vi "ROI entry-Previous ROI compat-planes.vi"(8 "error in (no error)":errorcluster, 9 "Proceed":bool=TRUE, 11 "Old ROI file path":path) -> (0 "error out":errorcluster, 1 "Proceed":bool, 3 "Old ROI file path (dup)":path)   [LabVIEW 2013]
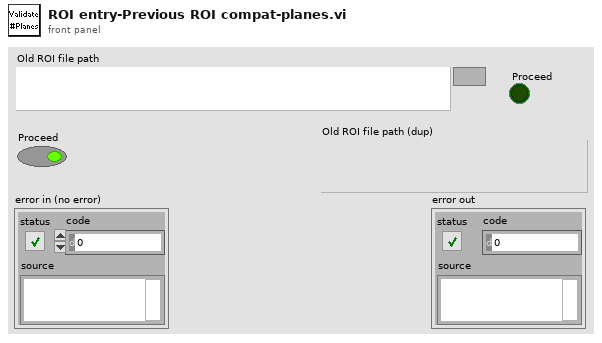
[diagram p1: front panel]
types:
  T1 = typedef "Fixed strings.ctl" = cluster{"ROI file name":string, "Normalised ROI file name":string, "Zplane Pockels values file name":string, "Functional data folder name":string, "Experiment Header file name":string, "Z-stack images folder name":string, "Groups setup rel. path":string, "Groups text file rel. path":string, "TDMS files folder name (F.img)":string, "TDMS files folder name (V.acq)":string, "TDMS files folder name (Pl.acq)":string, "Cycle rel times sequence file":string, "Dynamically called VIs folder name":string, "Time Series folder base name":string}
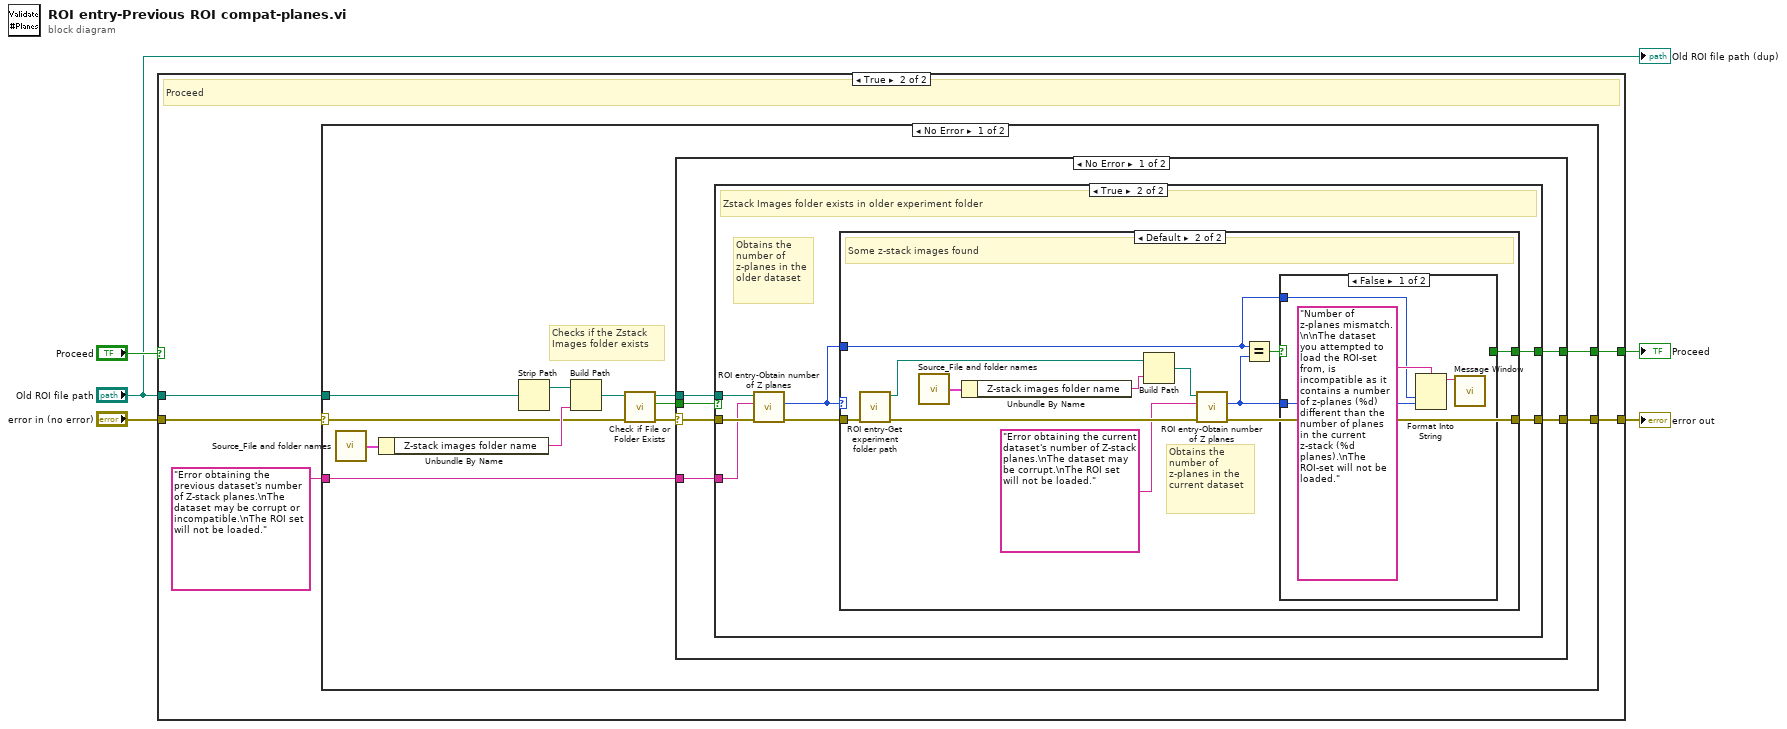
[diagram p0: block diagram]
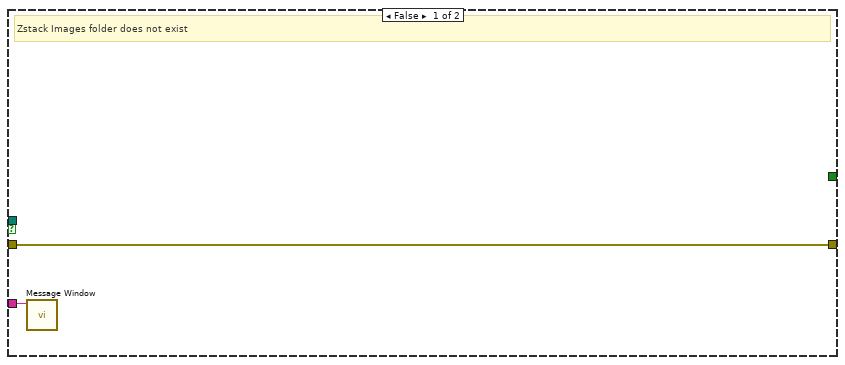
[diagram p3: hidden frame]
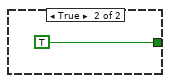
[diagram p5: hidden frame]
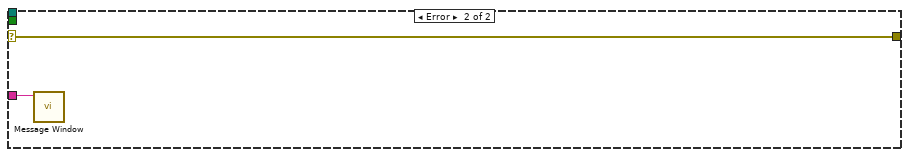
[diagram p6: hidden frame]
diagram:
  n1 = case shown="True" "Proceed" {
    tunnel: "Old ROI file path" -> [_ w11]
    tunnel: [w6 w9] -> w5
    tunnel: "error in (no error)" -> [w6 w8]
    tunnel: [_ w7] -> w3
    frame False {
      # "Skip"
    }
    frame True {
      # "Proceed"
      n2 = case shown="No Error" w8 {
        selector: w8 -> [w14 w59]
        tunnel: w11 -> [w21 _]
        tunnel: [w17 _] -> w7
        tunnel: [w13 w59] -> w9
        tunnel: "Error obtaining the previous dataset's number of Z-stack planes.\nThe dataset may be corrupt or incompatible.\nThe ROI set will not be loaded." ("Message string") -> [w12 _]
        frame No Error {
          # "Checks if the Zstack Images folder exists"
          n3 = call "Source_File and folder names.vi"() -> ("Fixed strings"=w22:T1)  [unwired: 1 in]
          n4 = Unbundle By Name(w22) -> ("Z-stack images folder name"=w19:string)
          n5 = Strip Path(path=w21) -> (stripped path=w20:path)  [unwired: 1 out]
          n6 = Build Path(base path=w20, name or relative path=w19) -> (appended path=w23:path)
          n7 = call <vilib>:"Check if File or Folder Exists.vi"("error in (no error)"=w14, "path"=w23) -> ("error out"=w15:errorcluster, "file or folder exists?"=w18:bool, "dup path"=w16:path)  [unwired: 7 in]
          n8 = case shown="No Error" w15 {
            selector: w15 -> [w26 w58]
            tunnel: w18 -> [w29 _]
            tunnel: [w28 _] -> w17
            tunnel: w16 -> [w27 _]
            tunnel: [w25 w58] -> w13
            tunnel: w12 -> [w24 w57]
            frame No Error {
              n9 = case shown="True" w29 {
                tunnel: [_ w32] -> w28
                tunnel: w27 -> [_ w38]
                tunnel: w26 -> [w31 w37]
                tunnel: [w31 w35] -> w25
                tunnel: w24 -> [w30 w34]
                frame False {
                  # "Zstack Images folder does not exist"
                  n10 = call "Message Window.vi"("Message string"=w30) -> ()  [unwired: 10 in, 1 out]
                }
                frame True {
                  # "Obtains the number of z-planes in the older dataset"
                  # "Zstack Images folder exists in older experiment folder"
                  n11 = call "ROI entry-Obtain number of Z planes.vi"("error in (no error)"=w37, "Message string"=w34, "Z-stack images folder path"=w38) -> ("error out"=w36:errorcluster, "Number of planes"=w33:i32)  [unwired: 6 in, 1 out]
                  n12 = case shown="Default" w33 {
                    tunnel: w36 -> [w39 w49]
                    tunnel: [w39 w46] -> w35
                    tunnel: w33 -> [_ w41]
                    tunnel: [_ w42] -> w32
                    frame 0 {
                      # "No z-stack images found"
                    }
                    frame Default {
                      # "Obtains the number of z-planes in the current dataset"
                      # "Some z-stack images found"
                      n13 = call "ROI entry-Get experiment folder path.vi"("error in (no error)"=w49) -> ("error out"=w47:errorcluster, "Experiment folder path"=w45:path)  [unwired: 9 in]
                      n14 = call "Source_File and folder names.vi"() -> ("Fixed strings"=w51:T1)  [unwired: 1 in]
                      n15 = Unbundle By Name(w51) -> ("Z-stack images folder name"=w50:string)
                      n16 = Build Path(base path=w45, name or relative path=w50) -> (appended path=w48:path)
                      n17 = call "ROI entry-Obtain number of Z planes.vi"("error in (no error)"=w47, "Message string"="Error obtaining the current dataset's number of Z-stack planes.\nThe dataset may be corrupt.\nThe ROI set will not be loaded.", "Z-stack images folder path"=w48) -> ("error out"=w46:errorcluster, "Number of planes"=w40:i32)  [unwired: 6 in, 1 out]
                      n18 = Equal?(x=w41, y=w40) -> (x = y?=w43:bool)
                      n19 = case shown="False" w43 {
                        tunnel: [_ TRUE] -> w42
                        tunnel: w41 -> [w53 _]
                        tunnel: w40 -> [w52 _]
                        frame False {
                          n20 = Format Into String(format string="Number of z-planes mismatch.\n\nThe dataset you attempted to load the ROI-set from, is incompatible as it contains a number of z-planes (%d) different than the number of planes in the current z-stack (%d planes).\nThe ROI-set will not be loaded." ("Message string"), w53, w52) -> (resulting string=w55:string)  [unwired: 2 in, 1 out]
                          n21 = call "Message Window.vi"("Message string"=w55) -> ()  [unwired: 10 in, 1 out]
                        }
                        frame True {
                        }
                      }
                    }
                  }
                }
              }
            }
            frame Error {
              n22 = call "Message Window.vi"("Message string"=w57) -> ()  [unwired: 10 in, 1 out]
            }
          }
        }
        frame Error {
        }
      }
    }
  }
  "error out" <- w5
  "Proceed" <- w3
  "Old ROI file path (dup)" <- "Old ROI file path"
